vi "AerotechScope.vi"(0 "error in (no error)":errorcluster) -> (3 "error out":errorcluster, 5 "AEROTECH.SCOPE":T1)   [LabVIEW 2009]
uses:
  Controls/AerotechScope.ctl
  Controls/AerotechCommand.ctl
  Controls/AerotechState.ctl
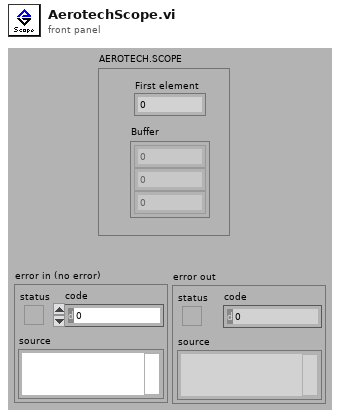
[diagram p1: front panel]
types:
  T1 = typedef "AerotechScope.ctl" = cluster{"First element":i32, "Buffer":i32[]}
  T2 = typedef "AerotechState.ctl" = enum16{"INITING", "IDLING", "SLEWING", "TRACKING", "MOVING", "HOMING", "STOPPING", "RECORDING"}
  T3 = typedef "AerotechCommand.ctl" = enum16{"TRACK", "POSITION", "STOP", "HOME", "QUIT", "RECORD"}
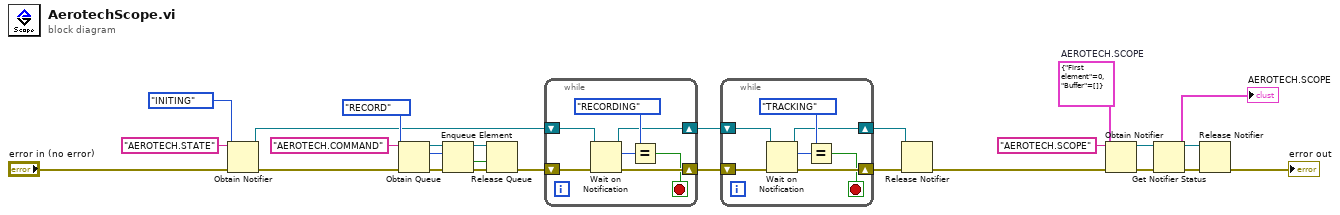
[diagram p0: block diagram]
diagram:
  w17 = AerotechCommand."RECORD" ("Command")
  w22 = T1 {"First element"=0, "Buffer"=[]}  # AEROTECH.SCOPE
  n1 = Obtain Notifier(name (unnamed)="AEROTECH.STATE", notification data type=AerotechState."INITING" ("State"), error in (no error)="error in (no error)") -> (notifier out=w1:refnum<notifier>, error out=w2:errorcluster)  [unwired: 1 in, 1 out]
  n2 = Obtain Queue(name (unnamed)="AEROTECH.COMMAND", element data type=w17, error in (no error)=w2) -> (queue out=w18:refnum<queue>, error out=w19:errorcluster)  [unwired: 2 in, 1 out]
  n3 = Enqueue Element(queue=w18, element=w17, error in (no error)=w19) -> (queue out=w15:refnum<queue>, timed out?=w16:bool, error out=w14:errorcluster)  [unwired: 1 in]
  n4 = Release Queue(queue=w15, force destroy? (F)=w16, error in (no error)=w14) -> (error out=w9:errorcluster)  [unwired: 2 out]
  n5 = while {
    shift-right: [w27] -> w8
    shift-left: w1 -> [w31]
    shift-right: [w32] -> w7
    shift-left: w9 -> [w33]
    stop <- w28 stop-if-true
    n6 = Wait on Notification(notifier=w31, error in (no error)=w33) -> (notifier out=w27:refnum<notifier>, notification=w30:T2, error out=w32:errorcluster)  [unwired: 2 in, 1 out]
    n7 = Equal?(x=AerotechState."RECORDING" ("notification"), y=w30) -> (x = y?=w28:bool)
  }
  n8 = while {
    shift-right: [w34] -> w4
    shift-left: w8 -> [w38]
    shift-right: [w39] -> w6
    shift-left: w7 -> [w40]
    stop <- w35 stop-if-true
    n9 = Wait on Notification(notifier=w38, error in (no error)=w40) -> (notifier out=w34:refnum<notifier>, notification=w37:T2, error out=w39:errorcluster)  [unwired: 2 in, 1 out]
    n10 = Equal?(x=AerotechState."TRACKING" ("notification"), y=w37) -> (x = y?=w35:bool)
  }
  n11 = Release Notifier(notifier=w4, error in (no error)=w6) -> (error out=w5:errorcluster)  [unwired: 1 in, 2 out]
  n12 = Obtain Notifier(name (unnamed)="AEROTECH.SCOPE", notification data type=w22, error in (no error)=w5) -> (notifier out=w13:refnum<notifier>, error out=w3:errorcluster)  [unwired: 1 in, 1 out]
  n13 = Get Notifier Status(notifier=w13, error in (no error)=w3) -> (notifier out=w24:refnum<notifier>, current notification=→"AEROTECH.SCOPE":T1, error out=w25:errorcluster)  [unwired: 2 out]
  n14 = Release Notifier(notifier=w24, error in (no error)=w25) -> (error out=→"error out":errorcluster)  [unwired: 1 in, 2 out]
